vi "User Operator Panel.vi"() -> ()   [LabVIEW 2026]
uses:
  Host State.ctl
  RT Commands.ctl
  Game Settings.ctl
  RT States.ctl
  Score.ctl
  SideSelector.ctl
  5b16e98e-8c62-4f4c-9228-1465c9ac843a.vi
  <extravilib>/ChannelInstances/Tag-bool/Read With Abort.vi
  <extravilib>/ChannelInstances/Tag-bool/Write With Abort.vi
  <extravilib>/ChannelInstances/Tag-bool/Instantiate.vi
  <extravilib>/ChannelInstances/Tag-bool/EndpointRead.vi
  <extravilib>/ChannelInstances/Tag-bool/Endpoint.vi
  <extravilib>/ChannelInstances/Tag-bool.lvlib
panel:
  in  "Button 1":bool
  in  "Player 1 Name":string
  in  "Button 2":bool
  in  "Player 2 Name":string
  out "Final Score":T1
  in  "GO":bool
  out "Status":string
  # "(Ctl+Shfit+GO! to terminate program)"
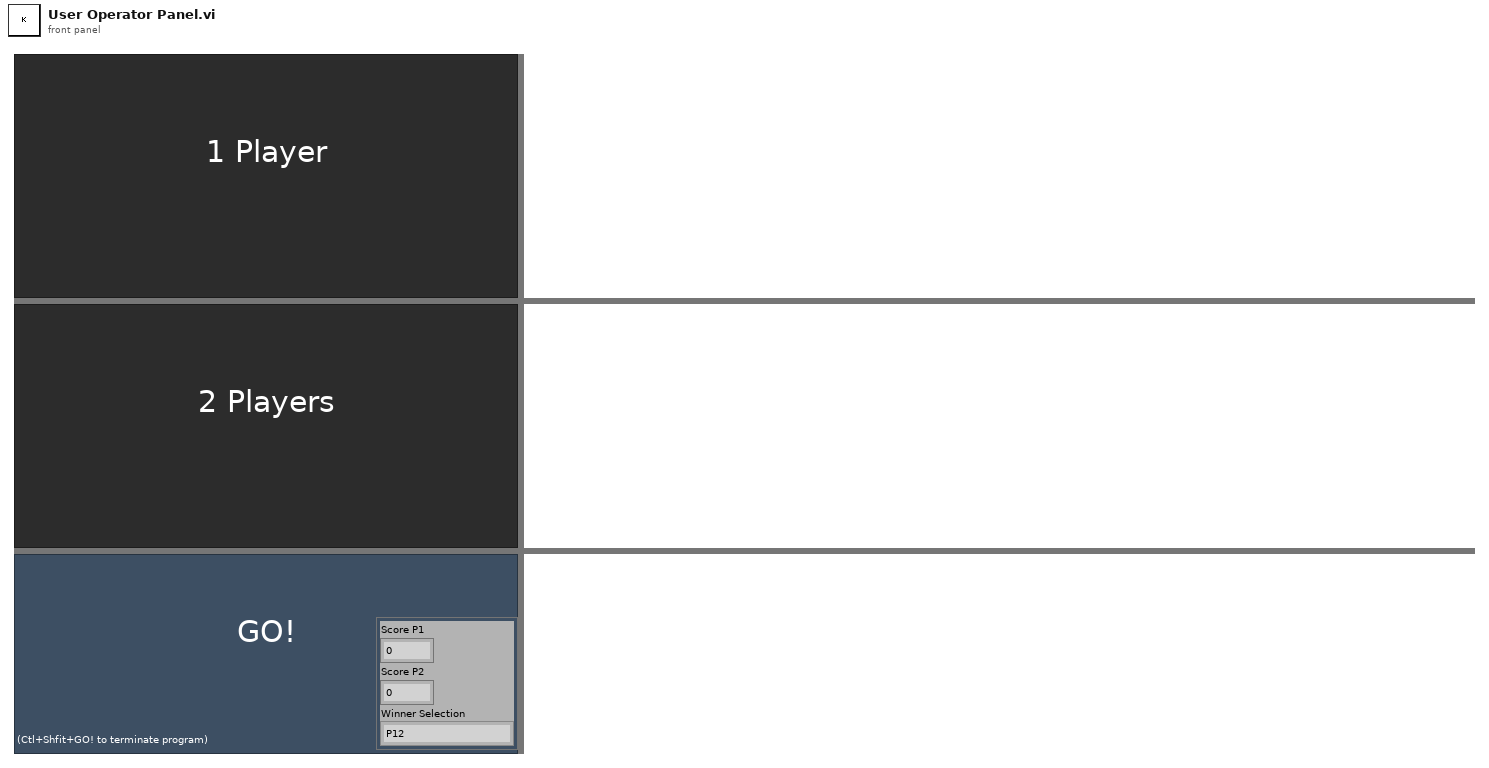
[diagram p1: front panel]
types:
  T1 = typedef "Score.ctl" = cluster{"Score P1":u16, "Score P2":u16, "Winner Selection":T2}
  T2 = typedef "SideSelector.ctl" = enum16{"P12", "P1", "P2"}
  T3 = typedef "Host State.ctl" = enum16{"<startup>", "Idle", "StartGame", "WaitForCompletion", "Announce Winner"}
  T4 = typedef "RT Commands.ctl" = enum16{"<null>", "End Idle", "Reset", "Commit Settings", "Commit Host Settings"}
  T5 = typedef "Game Settings.ctl" = cluster{"Speed Threshold, ticks":u64, "Game Time":u32, "2 Players":bool}
  T6 = typedef "RT States.ctl" = enum16{"Idle", "Configuring", "1Player", "2Player", "Display Winner"}
  T7 = typedef "Tag-bool.lvlib/))Channel.ctl" = refnum<queue>
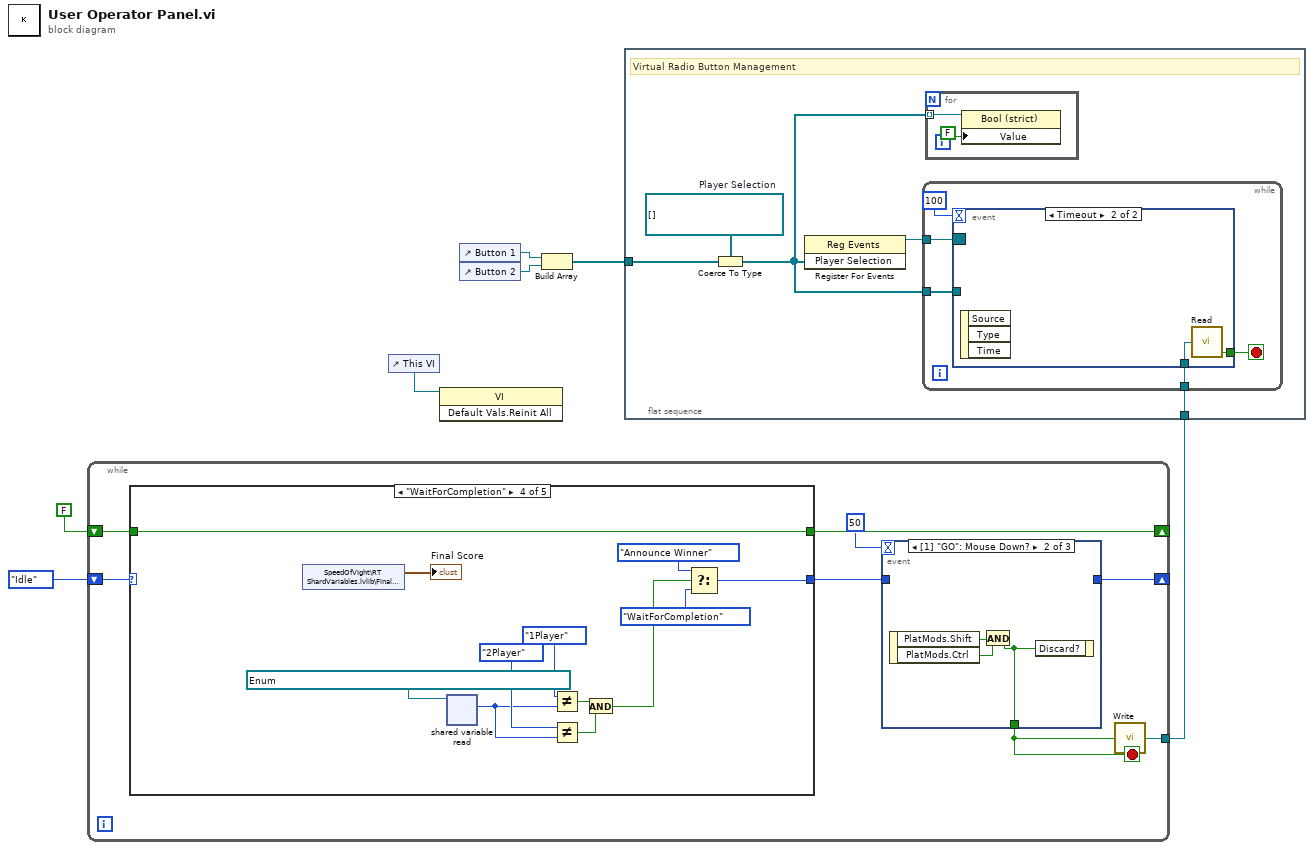
[diagram p0: block diagram]
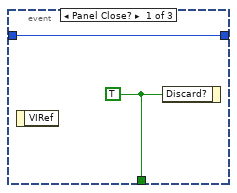
[diagram p2: hidden frame]
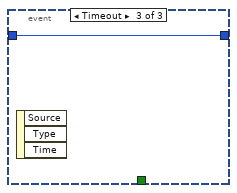
[diagram p3: hidden frame]
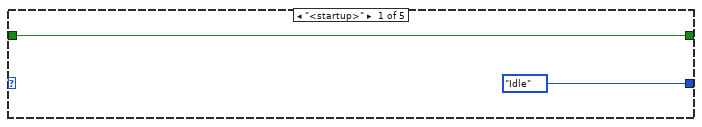
[diagram p4: hidden frame]
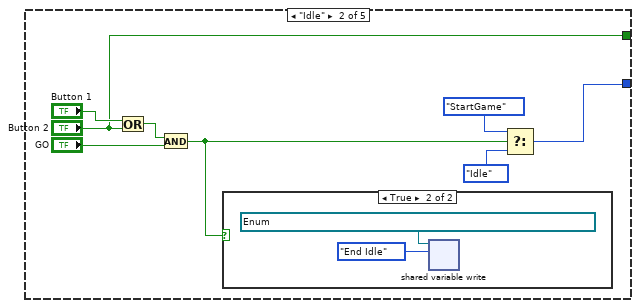
[diagram p5: hidden frame]
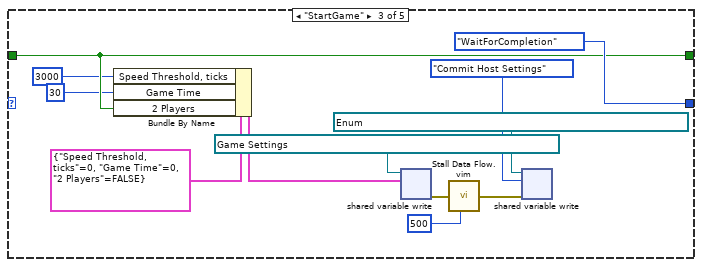
[diagram p7: hidden frame]
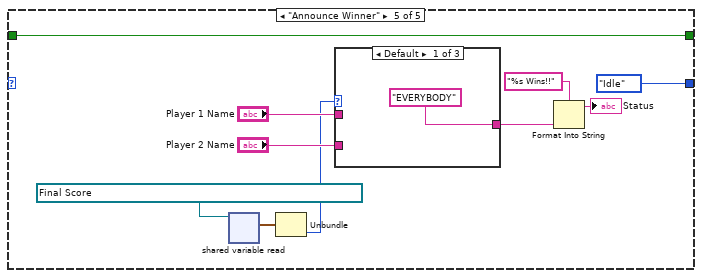
[diagram p8: hidden frame]
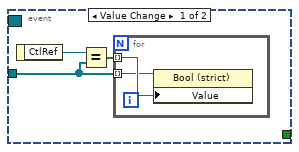
[diagram p11: hidden frame]
diagram:
  n1 = while {
    shift-right: [w10] -> _
    shift-left: Host_State."Idle" -> [w15]
    shift-right: [w14] -> _
    shift-left: FALSE ("Button 2") -> [w13]
    tunnel: [w8] -> w1
    stop <- w11 stop-if-true
    n2 = case shown="\"WaitForCompletion\"" w15 {
      tunnel: [Host_State."Idle" w31 Host_State."WaitForCompletion" w54 Host_State."Idle" ("f")] -> w12
      tunnel: [w22 "Button 2" w42 w57 w64] -> w14
      tunnel: w13 -> [w22 _ w42 w57 w64]
      frame "<startup>" {
      }
      frame "Idle" {
        n3 = Or(x="Button 1", y="Button 2") -> (x .or. y?=w26:bool)
        n4 = And(x=w26, y="GO") -> (x .and. y?=w24:bool)
        n5 = case shown="True" w24 {
          frame False {
          }
          frame True {
            w33 = refnum<k21> "ni.var.psp://SpeedOfVIght/RT ShardVariables/H2RTCommand" items=["<null>", "End Idle", "Reset", "Commit Settings", "Commit Host Settings"] ("shared variable refnum in")
            n6 = shared-variable-write(w33, RT_Commands."End Idle" ("H2RTCommand")) -> ()  [unwired: 1 in, 2 out]
          }
        }
        n7 = Select(t=Host_State."StartGame", s=w24, f=Host_State."Idle") -> (s? t:f=w31:T3)
      }
      frame "StartGame" {
        w37 = refnum<k21> "ni.var.psp://SpeedOfVIght/RT ShardVariables/H2RTCommand" items=["<null>", "End Idle", "Reset", "Commit Settings", "Commit Host Settings"] ("shared variable refnum in")
        n8 = Bundle By Name(cluster=T5 {"Speed Threshold, ticks"=0, "Game Time"=0, "2 Players"=FALSE} ("Game Settings"), "Speed Threshold, ticks"=u64 3000, "Game Time"=u32 30, "2 Players"=w42) -> (w43:T5)
        n9 = shared-variable-write(refnum<k21> "ni.var.psp://SpeedOfVIght/RT ShardVariables/Game Settings" ("shared variable refnum in"), w43) -> (w35:errorcluster)  [unwired: 1 in, 1 out]
        n10 = call "Stall Data Flow.vim"("value in"=w35, "milliseconds to wait"=u32 500) -> ("value out"=w34:errorcluster)  [unwired: 1 out]
        n11 = shared-variable-write(w37, w34, RT_Commands."Commit Host Settings" ("H2RTCommand")) -> ()  [unwired: 2 out]
      }
      frame "WaitForCompletion" {
        w56 = refnum<k21> "ni.var.psp://SpeedOfVIght/RT ShardVariables/RT2HState" items=["Idle", "Configuring", "1Player", "2Player", "Display Winner"] ("shared variable refnum in")
        n12 = shared-variable "SpeedOfVIght\\RT ShardVariables.lvlib\\Final Score"() -> (→"Final Score":T1)  [unwired: 1 in, 1 out]
        n13 = shared-variable-read(w56) -> (w49:T6)  [unwired: 1 in, 2 out]
        n14 = Not Equal?(x=RT_States."1Player", y=w49) -> (x != y?=w53:bool)
        n15 = Not Equal?(x=RT_States."2Player", y=w49) -> (x != y?=w48:bool)
        n16 = And(x=w53, y=w48) -> (x .and. y?=w47:bool)
        n17 = Select(t=Host_State."Announce Winner", s=w47, f=Host_State."WaitForCompletion") -> (s? t:f=w54:T3)
      }
      frame "Announce Winner" {
        n18 = shared-variable-read(refnum<k21> "ni.var.psp://SpeedOfVIght/RT ShardVariables/Final Score" ("shared variable refnum in")) -> (w62:T1)  [unwired: 1 in, 2 out]
        n19 = Unbundle(w62) -> ("Winner Selection"=w58:T2)  [unwired: 2 out]
        n20 = case shown="Default" w58 {
          tunnel: ["EVERYBODY" ("Player 1 Name") w69 w70] -> w61
          tunnel: "Player 1 Name" -> [_ w69 _]
          tunnel: "Player 2 Name" -> [_ _ w70]
          frame Default {
          }
          frame "P1" {
          }
          frame "P2" {
          }
        }
        n21 = Format Into String(format string="%s Wins!!", w61) -> (resulting string=→"Status":string)  [unwired: 2 in, 1 out]
      }
    }
    n22 = event shown="[1] \"GO\": Mouse Down?" {
      selector: _ -> [_ _ _]
      dyn-events: _ -> [_ _ _]
      timeout: 50 -> [_ _ _]
      tunnel: w12 -> [w16 _ w21]
      tunnel: [w17 w18 _] -> w11
      tunnel: [w16 _ w21] -> w10
      event Panel Close? {
        w17 = TRUE ("Discard?")
        n23 = event-data() -> ()  [unwired: 1 in, 1 out]
        n24 = event-data("Discard?"=w17) -> ()  [unwired: 1 in, 1 out]
      }
      event "GO": Mouse Down? {
        n25 = event-data() -> ("PlatMods.Shift"=w20:bool, "PlatMods.Ctrl"=w19:bool)  [unwired: 1 in]
        n26 = And(x=w20, y=w19) -> (x .and. y?=w18:bool)
        n27 = event-data("Discard?"=w18) -> ()  [unwired: 1 in, 1 out]
      }
      event Timeout {
        n28 = event-data() -> ()  [unwired: 1 in, 3 out]
      }
    }
    n29 = call <extravilib>:"Write.vi"("element"=w11) -> ("channel"=w8:T7)  [unwired: 1 out]
  }
  n30 = control-ref of="This VI"() -> (w2:refnum<vi>)
  n31 = invoke class="VI" method="Default Vals.Reinit All"(reference=w2) -> ()  [unwired: 2 in, 3 out]
  n32 = control-ref of="Button 1"() -> (w7:refnum<vi>)
  n33 = control-ref of="Button 2"() -> (w6:refnum<vi>)
  n34 = Build Array(w7, w6) -> (w5:refnum<vi>[])
  n35 = flat-sequence {
    tunnel: w5 -> [w74]
    tunnel: w1 -> [w71]
    frame #0 {
      w72 = refnum<vi>[] []  # Player Selection
      # "Virtual Radio Button Management"
      n36 = Coerce To Type(0:w74, 1:w72) -> (2:w73:refnum<vi>[])
      n37 = register-events(w73) -> (reference out=w75:refnum<event-registration>)  [unwired: 2 in, 1 out]
      n38 = while {
        tunnel: w75 -> [w82]
        tunnel: w73 -> [w81]
        tunnel: w71 -> [w78]
        stop <- w80 stop-if-true
        n39 = event shown="[1] Timeout" {
          selector: w82 -> [_ _]
          dyn-events: _ -> [_ _]
          timeout: 100 -> [_ _]
          tunnel: w81 -> [w83 _]
          tunnel: [_ w88] -> w80
          tunnel: w78 -> [_ w89]
          event Value Change {
            n40 = event-data() -> ("CtlRef"=w85:refnum<vi>)  [unwired: 1 in]
            n41 = Equal?(x=w85, y=w83) -> (x = y?=w84:bool[])
            n42 = for {
              tunnel: w84 -> [w87] mode=indexing
              tunnel: w83 -> [w86] mode=indexing
              n43 = property class="Bool (strict)"(reference=w86, "Value"=w87) -> ()  [unwired: 1 in, 2 out]
            }
          }
          event Timeout {
            n44 = event-data() -> ()  [unwired: 1 in, 3 out]
            n45 = call <extravilib>:"Read.vi"("channel"=w89) -> ("element"=w88:bool)  [unwired: 1 in, 1 out]
          }
        }
      }
      n46 = for {
        tunnel: w73 -> [w77] mode=indexing
        n47 = property class="Bool (strict)"(reference=w77, "Value"=FALSE) -> ()  [unwired: 1 in, 2 out]
      }
    }
  }
